vi "imaqrio_DownloadMethImpl.vi"(4 "error in (no error)":errorcluster, 5 "vi path":path, 6 "Force Download (F)":bool, 7 "HW Exec Ref":refnum<visa-resource-name>) -> (0 "error out":errorcluster, 3 "HW Exec Ref (Dup)":refnum<visa-resource-name>)   [LabVIEW 2017]
doc: "This VI will force a download to the FPGA board."
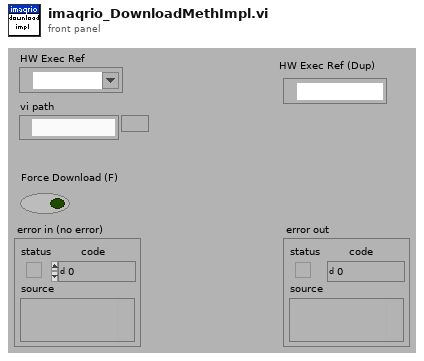
[diagram p1: front panel]
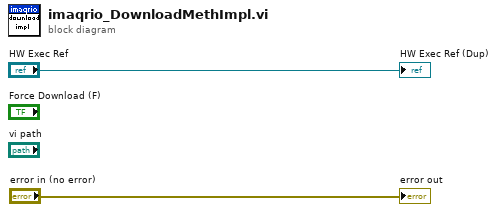
[diagram p0: block diagram]
diagram:
  "error out" <- "error in (no error)"
  "HW Exec Ref (Dup)" <- "HW Exec Ref"
